vi "update.vi"(8 "error in (no error)":errorcluster, 10 "update":refnum<class "GenericImageProcessor.lvclass">, 11 "DL090216RangeOffsetImageProcessor in":refnum<class "ImageProcessorDL090216RangeOffset.lvclass">) -> (0 "error out":errorcluster, 3 "DL090216RangeOffsetImageProcessor out":refnum<class "ImageProcessorDL090216RangeOffset.lvclass">)   [LabVIEW 2010, in "ImageProcessorDL090216RangeOffset.lvclass"]
uses:
  ImageProcessorDL090216RangeOffset.lvclass
  GenericImageProcessor/GenericImageProcessor/GenericImageProcessor.lvclass
  ImageProcessorDL090216RangeOffset.lvclass/ImageProcessorDL090216RangeOffset.ctl
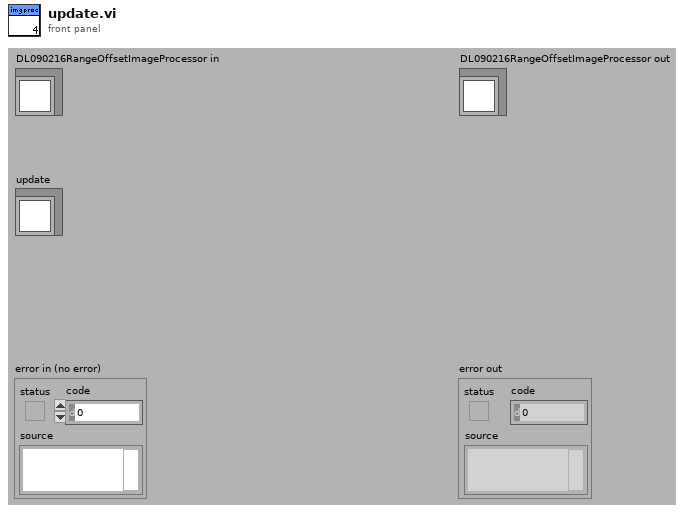
[diagram p1: front panel]
types:
  T1 = typedef "range_offset_cluster.ctl" = cluster{"range":dbl, "offset":dbl}
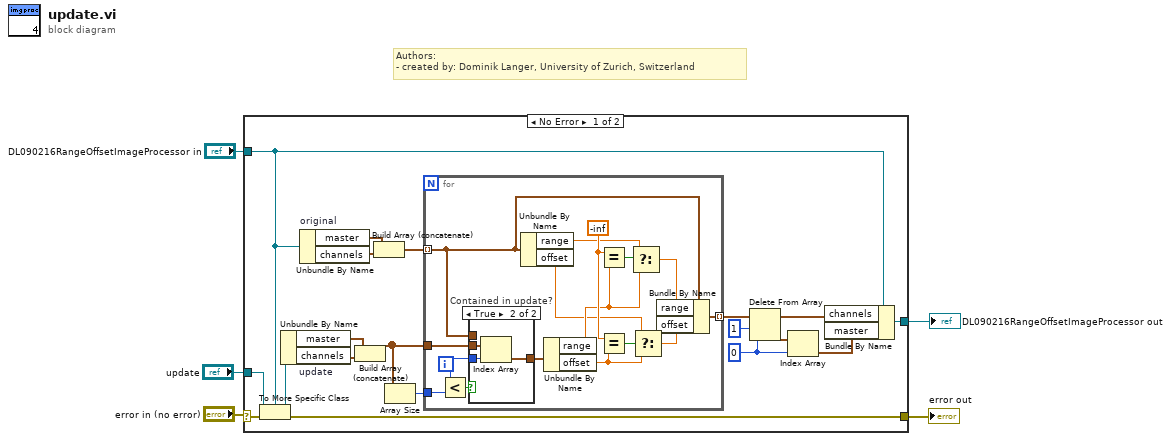
[diagram p0: block diagram]
diagram:
  # "Authors: \n- created by: Dominik Langer, University of Zurich, Switzerland"
  n1 = case shown="No Error" "error in (no error)" {
    selector: "error in (no error)" -> [w23 w46]
    tunnel: [w22 w46] -> w4
    tunnel: [w20 w45] -> w2
    tunnel: "DL090216RangeOffsetImageProcessor in" -> [w19 w45]
    tunnel: "update" -> [w24 _]
    frame No Error {
      w9 = 0 ("index")
      n2 = To More Specific Class(target class=w19, reference=w24, error in=w23) -> (specific class reference=w21:refnum<class "ImageProcessorDL090216RangeOffset.lvclass">, error out=w22:errorcluster)
      n3 = Unbundle By Name "update"(w21) -> ("master"=w15:T1, "channels"=w14:T1[])
      n4 = Unbundle By Name "original"(w19) -> ("master"=w17:T1, "channels"=w18:T1[])
      n5 = Build Array (concatenate)(w15, w14) -> (w7:T1[])
      n6 = Build Array (concatenate)(w17, w18) -> (w16:T1[])
      n7 = Array Size(array=w7) -> (size(s)=w6:i32)
      n8 = for {
        tunnel: w16 -> [w25] mode=indexing
        tunnel: [w31] -> w13 mode=indexing
        tunnel: w7 -> [w29]
        tunnel: w6 -> [w28]
        i -> [w26]
        w39 = -inf
        n9 = Less?(x=w26, y=w28) -> (x < y?=w27:bool)
        n10 = case "Contained in update?" shown="True" w27 {
          tunnel: [w41 w44] -> w30
          tunnel: w29 -> [_ w43]
          tunnel: w26 -> [_ w42]
          tunnel: w25 -> [w41 _]
          frame False {
          }
          frame True {
            n11 = Index Array(array=w43, index=w42) -> (element=w44:T1)
          }
        }
        n12 = Unbundle By Name(w25) -> ("range"=w35:dbl, "offset"=w34:dbl)
        n13 = Unbundle By Name(w30) -> ("range"=w36:dbl, "offset"=w37:dbl)
        n14 = Equal?(x=w39, y=w36) -> (x = y?=w38:bool)
        n15 = Equal?(x=w39, y=w37) -> (x = y?=w40:bool)
        n16 = Select(t=w35, s=w38, f=w36) -> (s? t:f=w33:dbl)
        n17 = Select(t=w34, s=w40, f=w37) -> (s? t:f=w32:dbl)
        n18 = Bundle By Name(cluster=w25, "range"=w33, "offset"=w32) -> (w31:T1)
      }
      n19 = Delete From Array(array=w13, length=1, index=w9) -> (deleted portion=w10:T1[], array with subset deleted=w11:T1[])
      n20 = Index Array(array=w10, index=w9) -> (element=w8:T1)
      n21 = Bundle By Name(cluster=w19, "channels"=w11, "master"=w8) -> (w20:refnum<class "ImageProcessorDL090216RangeOffset.lvclass">)
    }
    frame Error {
    }
  }
  "error out" <- w4
  "DL090216RangeOffsetImageProcessor out" <- w2
